vi "Configure.vi"(8 "error in (no error)":errorcluster, 11 "LineCCD in":refnum<class "LineCCD.lvclass">) -> (0 "error out":errorcluster, 2 "cancelled?":bool, 3 "LineCCD out":refnum<class "LineCCD.lvclass">)   [LabVIEW 2012, in "LineCCD.lvclass"]
doc: "The configure method configures the details for the RabbitMQ connection, the observers and the mapping script.\n\nIn the derived class, make a call to the parent for setting these parameters."
uses:
  LineCCD.lvclass
  <vilib>/Utility/miscctls.llb/LVPointTypeDef.ctl
  <vilib>/Distrio/Murmex/Murmex/Murmex.lvclass
  LineCCD.lvclass/LineCCD.ctl
panel:
  in  "button:ok":bool
  in  "button:cancel":bool
  in  "Tab Control":enum32{"LineCCD", "Page 2"}(tab)
  in  "Include dummy pixels in readouts":bool
  in  "Device Serial Number":string
  in  "Skip default setup":bool
  in  "button:call parent":bool
  # "RabbitMQ parameters"
  # "Window position"
  # "Sends a setting or configuration value to an observer, e.g. observer.parameter=settingsname;"
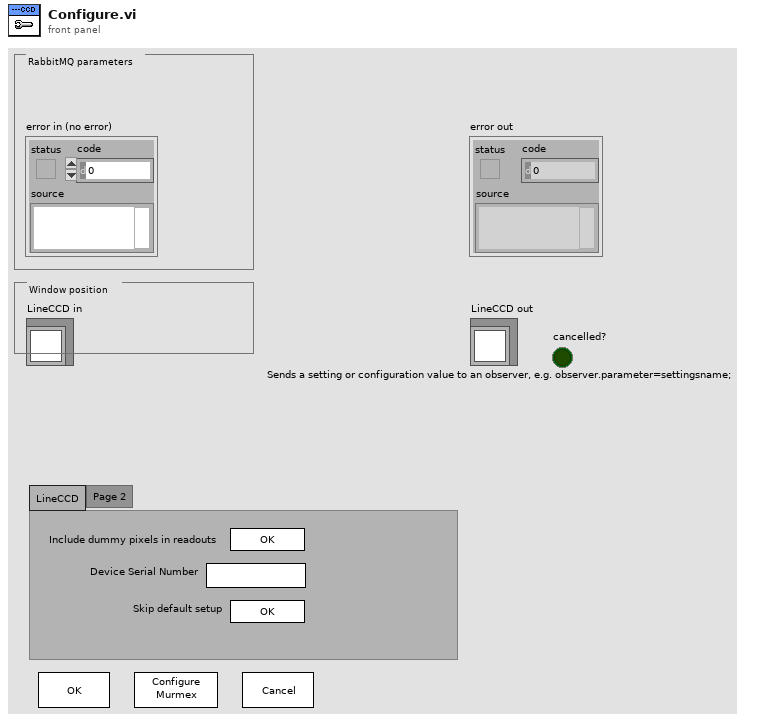
[diagram p1: front panel]
types:
  T1 = typedef "LVPointTypeDef.ctl" = cluster{"Horizontal":i16, "Vertical":i16}
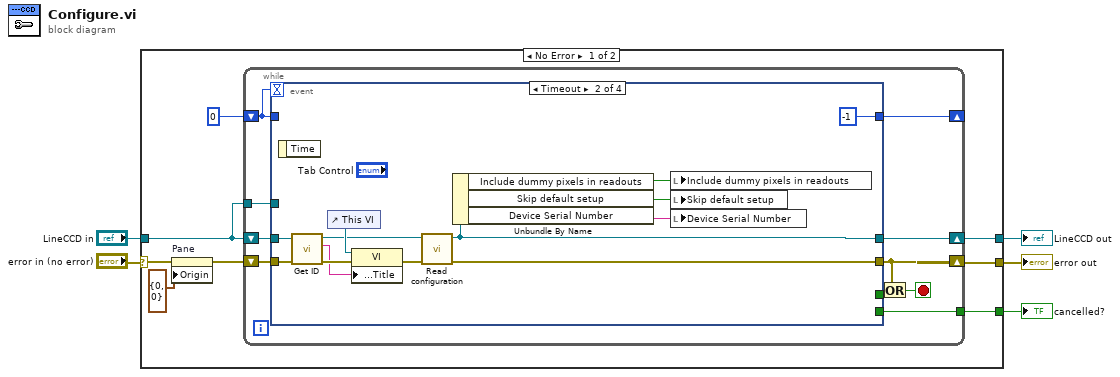
[diagram p0: block diagram]
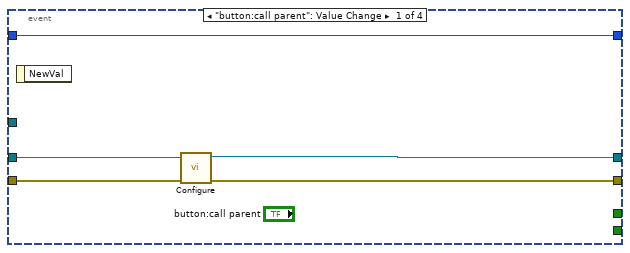
[diagram p2: hidden frame]
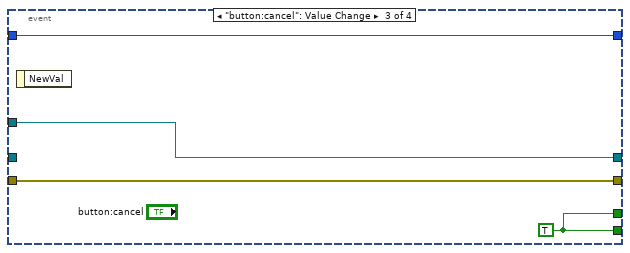
[diagram p3: hidden frame]
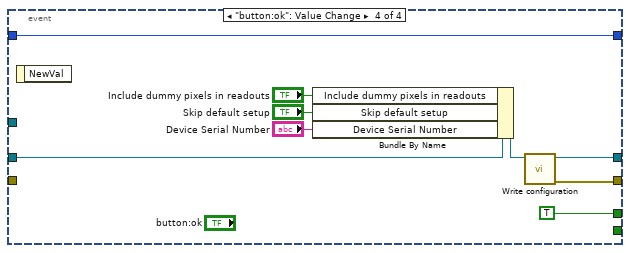
[diagram p4: hidden frame]
diagram:
  n1 = case shown="No Error" "error in (no error)" {
    selector: "error in (no error)" -> [w12 w55]
    tunnel: "LineCCD in" -> [w11 w56]
    tunnel: [w8 w56] -> w3
    tunnel: [w7 w55] -> w2
    tunnel: [w6 _] -> w1
    frame No Error {
      n2 = property on="Pane" class="Pane"(error in=w12, "Origin"=T1 {"Horizontal"=0, "Vertical"=0}) -> (error out=w10:errorcluster)  [unwired: 1 in, 1 out]
      n3 = while {
        tunnel: w11 -> [w15]
        shift-right: [w19] -> w7
        shift-left: w10 -> [w23]
        shift-right: [w20] -> w8
        shift-left: w11 -> [w22]
        shift-right: [w16] -> _
        shift-left: 0 -> [w21]
        tunnel: [w17] -> w6
        stop <- w18 stop-if-true
        n4 = event shown="[1] Timeout" {
          selector: _ -> [_ _ _ _]
          dyn-events: _ -> [_ _ _ _]
          timeout: w21 -> [_ _ _ _]
          tunnel: w23 -> [w28 w40 w44 _]
          tunnel: w22 -> [w27 w38 _ w50]
          tunnel: w21 -> [w24 _ w42 w53]
          tunnel: [w26 w33 w44 w52] -> w19
          tunnel: [w25 w32 w45 w51] -> w20
          tunnel: [_ _ w43 _] -> w17
          tunnel: [w24 -1 w42 w53] -> w16
          tunnel: w15 -> [_ _ w45 _]
          tunnel: [_ _ w43 TRUE ("cancelled?")] -> w14
          event "button:call parent": Value Change {
            n5 = event-data() -> ()  [unwired: 1 in, 1 out]
            n6 = call-parent "Configure.vi"("error in (no error)"=w28, "Murmex in"=w27) -> ("error out"=w26:errorcluster, "Murmex out"=w25:refnum<class "LineCCD.lvclass">)  [unwired: 7 in, 1 out]
          }
          event Timeout {
            n7 = event-data() -> ()  [unwired: 1 in, 1 out]
            n8 = call <vilib>:"Get ID.vi"("error in (no error)"=w40, "Murmex in"=w38) -> ("error out"=w39:errorcluster, "component id"=w37:string, "Murmex out"=w34:refnum<class "LineCCD.lvclass">)  [unwired: 7 in]
            n9 = control-ref of="This VI"() -> (w36:refnum<vi>)
            n10 = property class="VI"(reference=w36, error in=w39, "Front Panel.Title"=w37) -> (error out=w35:errorcluster)  [unwired: 1 out]
            n11 = call <vilib>:"Read configuration.vi"("error in (no error)"=w35, "Murmex in"=w34) -> ("error out"=w33:errorcluster, "Murmex out"=w32:refnum<class "LineCCD.lvclass">)  [unwired: 7 in, 1 out]
            n12 = Unbundle By Name(w32) -> ("Include dummy pixels in readouts"=w29:bool, "Skip default setup"=w30:bool, "Device Serial Number"=w31:string)
            n13 = local write "Include dummy pixels in readouts"(w29) -> ()
            n14 = local write "Skip default setup"(w30) -> ()
            n15 = local write "Device Serial Number"(w31) -> ()
          }
          event "button:cancel": Value Change {
            w43 = TRUE ("cancelled?")
            n16 = event-data() -> ()  [unwired: 1 in, 1 out]
          }
          event "button:ok": Value Change {
            n17 = event-data() -> ()  [unwired: 1 in, 1 out]
            n18 = Bundle By Name(cluster=w50, "Include dummy pixels in readouts"="Include dummy pixels in readouts", "Skip default setup"="Skip default setup", "Device Serial Number"="Device Serial Number") -> (w49:refnum<class "LineCCD.lvclass">)
            n19 = call <vilib>:"Write configuration.vi"("Murmex in"=w49) -> ("error out"=w52:errorcluster, "Murmex out"=w51:refnum<class "LineCCD.lvclass">)  [unwired: 9 in]
          }
        }
        n20 = Or(x=w19, y=w14) -> (x .or. y?=w18:bool)
      }
    }
    frame Error {
    }
  }
  "error out" <- w2
  "LineCCD out" <- w3
  "cancelled?" <- w1
